vi "prova connessione sql.vi"() -> ()   [LabVIEW 2016]
uses:
  <vilib>/addons/database/NI_Database_API.lvlib
  <vilib>/addons/database/Connection.llb/DB Tools Open Connec (String).vi
  <vilib>/addons/database/Connection.llb/Conn Set Properties.vi
panel:
  out "tables":string[](array[string])
  in  "string":string="Provider=SQLNCLI11.1;Integrated Security=SSPI;Persist Security Info=False;User ID=\"\";Initial Catalog=PUMPTEST_COLLAUDI;Data Source=TECNICO4\\SQLEXPRESS;Initial File Name=\"\";Server SPN=\"\""
  in  "password":string
  in  "userID":string
  in  "prompt? (F)":bool
  out "error out":errorcluster
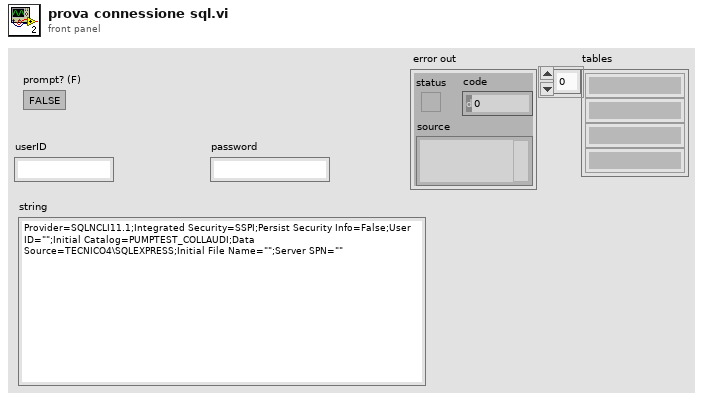
[diagram p1: front panel]
types:
  T1 = typedef "NI_Database_API.lvlib/Conn ObjectReference.ctl" = refnum<k1>
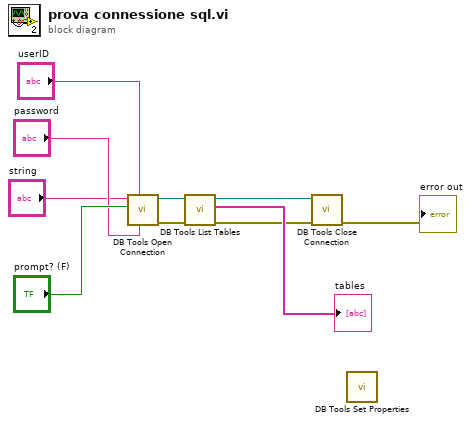
[diagram p0: block diagram]
diagram:
  n1 = call-poly <vilib>:"DB Tools Open Connection.vi"("password"="password", "userID"="userID", "prompt? (F)"="prompt? (F)", "connection information"="string") -> ("error out"=w2:errorcluster, "connection reference"=w5:T1)  [unwired: 4 in]
  n2 = call <vilib>:"DB Tools List Tables.vi"("error in (no error)"=w2, "connection reference"=w5) -> ("error out"=w1:errorcluster, "tables"=→"tables":string[], "connection reference out"=w3:T1)  [unwired: 3 in]
  "error out" <- w1
  n3 = call <vilib>:"DB Tools Close Connection.vi"("error in (no error)"=w1, "connection reference"=w3) -> ()  [unwired: 5 in, 1 out]
  n4 = call-poly <vilib>:"DB Tools Set Properties.vi"() -> ()  [unwired: 6 in, 2 out]
